vi "bit letters.vi"(8 "String \"0\"":string=" ", 9 "String \"1\"":string="#", 10 "Letras y string \"0\" / String \"1 y 0\"":bool=TRUE, 11 "Texto":string="Hola") -> (3 "big letters":string)   [LabVIEW 2019]
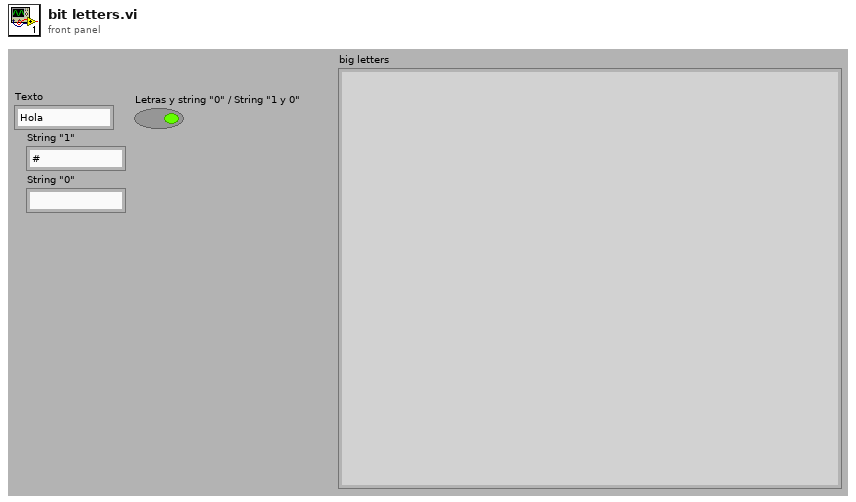
[diagram p1: front panel]
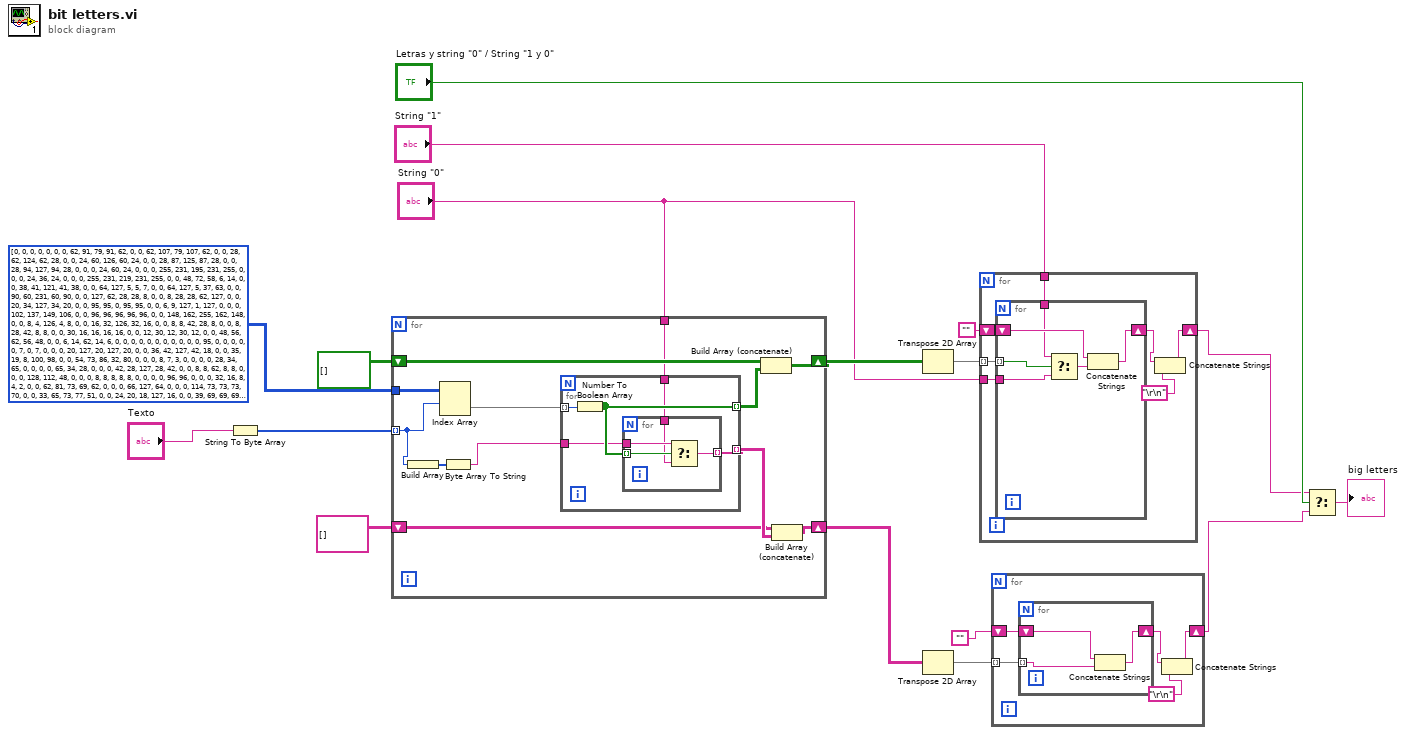
[diagram p0: block diagram]
diagram:
  n1 = String To Byte Array(string="Texto") -> (unsigned byte array=w16:u8[])
  n2 = for {
    tunnel: w16 -> [w24] mode=indexing
    tunnel: u8[][] [[0, 0, 0, 0, 0, 0, 0], [62, 91, 79, 91, 62, 0, 0], [62, 107, 79, 107, 62, 0, 0], [28, 62, 124, 62, 28, 0, 0], [24, 60, 126, 60, 24, 0, 0], [28, 87, 125, 87, 28, 0, 0], [28, 94, 127, 94, 28, 0, 0], [0, 24, 60, 24, 0, 0, 0], [255, 231, 195, 231, 255, 0, 0], [0, 24, 36, 24, 0, 0, 0], [255, 231, 219, 231, 255, 0, 0], [48, 72, 58, 6, 14, 0, 0], [38, 41, 121, 41, 38, 0, 0], [64, 127, 5, 5, 7, 0, 0], [64, 127, 5, 37, 63, 0, 0], [90, 60, 231, 60, 90, 0, 0], [127, 62, 28, 28, 8, 0, 0], [8, 28, 28, 62, 127, 0, 0], [20, 34, 127, 34, 20, 0, 0], [95, 95, 0, 95, 95, 0, 0], [6, 9, 127, 1, 127, 0, 0], [0, 102, 137, 149, 106, 0, 0], [96, 96, 96, 96, 96, 0, 0], [148, 162, 255, 162, 148, 0, 0], [8, 4, 126, 4, 8, 0, 0], [16, 32, 126, 32, 16, 0, 0], [8, 8, 42, 28, 8, 0, 0], [8, 28, 42, 8, 8, 0, 0], [30, 16, 16, 16, 16, 0, 0], [12, 30, 12, 30, 12, 0, 0], [48, 56, 62, 56, 48, 0, 0], [6, 14, 62, 14, 6, 0, 0], [0, 0, 0, 0, 0, 0, 0], [0, 0, 95, 0, 0, 0, 0], [0, 7, 0, 7, 0, 0, 0], [20, 127, 20, 127, 20, 0, 0], [36, 42, 127, 42, 18, 0, 0], [35, 19, 8, 100, 98, 0, 0], [54, 73, 86, 32, 80, 0, 0], [0, 8, 7, 3, 0, 0, 0], [0, 28, 34, 65, 0, 0, 0], [0, 65, 34, 28, 0, 0, 0], [42, 28, 127, 28, 42, 0, 0], [8, 8, 62, 8, 8, 0, 0], [0, 128, 112, 48, 0, 0, 0], [8, 8, 8, 8, 8, 0, 0], [0, 0, 96, 96, 0, 0, 0], [32, 16, 8, 4, 2, 0, 0], [62, 81, 73, 69, 62, 0, 0], [0, 66, 127, 64, 0, 0, 0], [114, 73, 73, 73, 70, 0, 0], [33, 65, 73, 77, 51, 0, 0], [24, 20, 18, 127, 16, 0, 0], [39, 69, 69, 69, 57, 0, 0], [60, 74, 73, 73, 49, 0, 0], [65, 33, 17, 9, 7, 0, 0], [54, 73, 73, 73, 54, 0, 0], [70, 73, 73, 41, 30, 0, 0], [0, 0, 20, 0, 0, 0, 0], [0, 64, 52, 0, 0, 0, 0], [0, 8, 20, 34, 65, 0, 0], [20, 20, 20, 20, 20, 0, 0], [0, 65, 34, 20, 8, 0, 0], [2, 1, 89, 9, 6, 0, 0], [62, 65, 93, 89, 78, 0, 0], [124, 18, 17, 18, 124, 0, 0], [127, 73, 73, 73, 54, 0, 0], [62, 65, 65, 65, 34, 0, 0], [127, 65, 65, 65, 62, 0, 0], [127, 73, 73, 73, 65, 0, 0], [127, 9, 9, 9, 1, 0, 0], [62, 65, 65, 81, 115, 0, 0], [127, 8, 8, 8, 127, 0, 0], [0, 65, 127, 65, 0, 0, 0], [32, 64, 65, 63, 1, 0, 0], [127, 8, 20, 34, 65, 0, 0], [127, 64, 64, 64, 64, 0, 0], [127, 2, 28, 2, 127, 0, 0], [127, 4, 8, 16, 127, 0, 0], [62, 65, 65, 65, 62, 0, 0], [127, 9, 9, 9, 6, 0, 0], [62, 65, 81, 33, 94, 0, 0], [127, 9, 25, 41, 70, 0, 0], [38, 73, 73, 73, 50, 0, 0], [3, 1, 127, 1, 3, 0, 0], [63, 64, 64, 64, 63, 0, 0], [31, 32, 64, 32, 31, 0, 0], [63, 64, 56, 64, 63, 0, 0], [99, 20, 8, 20, 99, 0, 0], [3, 4, 120, 4, 3, 0, 0], [97, 89, 73, 77, 67, 0, 0], [0, 127, 65, 65, 65, 0, 0], [2, 4, 8, 16, 32, 0, 0], [0, 65, 65, 65, 127, 0, 0], [4, 2, 1, 2, 4, 0, 0], [64, 64, 64, 64, 64, 0, 0], [0, 3, 7, 8, 0, 0, 0], [32, 84, 84, 120, 64, 0, 0], [127, 40, 68, 68, 56, 0, 0], [56, 68, 68, 68, 40, 0, 0], [56, 68, 68, 40, 127, 0, 0], [56, 84, 84, 84, 24, 0, 0], [0, 8, 126, 9, 2, 0, 0], [24, 164, 164, 156, 120, 0, 0], [127, 8, 4, 4, 120, 0, 0], [0, 68, 125, 64, 0, 0, 0], [32, 64, 64, 61, 0, 0, 0], [127, 16, 40, 68, 0, 0, 0], [0, 65, 127, 64, 0, 0, 0], [124, 4, 120, 4, 120, 0, 0], [124, 8, 4, 4, 120, 0, 0], [56, 68, 68, 68, 56, 0, 0], [252, 24, 36, 36, 24, 0, 0], [24, 36, 36, 24, 252, 0, 0], [124, 8, 4, 4, 8, 0, 0], [72, 84, 84, 84, 36, 0, 0], [4, 4, 63, 68, 36, 0, 0], [60, 64, 64, 32, 124, 0, 0], [28, 32, 64, 32, 28, 0, 0], [60, 64, 48, 64, 60, 0, 0], [68, 40, 16, 40, 68, 0, 0], [76, 144, 144, 144, 124, 0, 0], [68, 100, 84, 76, 68, 0, 0], [0, 8, 54, 65, 0, 0, 0], [0, 0, 119, 0, 0, 0, 0], [0, 65, 54, 8, 0, 0, 0], [2, 1, 2, 4, 2, 0, 0], [60, 38, 35, 38, 60, 0, 0], [30, 161, 161, 97, 18, 0, 0], [58, 64, 64, 32, 122, 0, 0], [56, 84, 84, 85, 89, 0, 0], [33, 85, 85, 121, 65, 0, 0], [33, 84, 84, 120, 65, 0, 0], [33, 85, 84, 120, 64, 0, 0], [32, 84, 85, 121, 64, 0, 0], [12, 30, 82, 114, 18, 0, 0], [57, 85, 85, 85, 89, 0, 0], [57, 84, 84, 84, 89, 0, 0], [57, 85, 84, 84, 88, 0, 0], [0, 0, 69, 124, 65, 0, 0], [0, 2, 69, 125, 66, 0, 0], [0, 1, 69, 124, 64, 0, 0], [240, 41, 36, 41, 240, 0, 0], [240, 40, 37, 40, 240, 0, 0], [124, 84, 85, 69, 0, 0, 0], [32, 84, 84, 124, 84, 0, 0], [124, 10, 9, 127, 73, 0, 0], [50, 73, 73, 73, 50, 0, 0], [50, 72, 72, 72, 50, 0, 0], [50, 74, 72, 72, 48, 0, 0], [58, 65, 65, 33, 122, 0, 0], [58, 66, 64, 32, 120, 0, 0], [0, 157, 160, 160, 125, 0, 0], [57, 68, 68, 68, 57, 0, 0], [61, 64, 64, 64, 61, 0, 0], [60, 36, 255, 36, 36, 0, 0], [72, 126, 73, 67, 102, 0, 0], [43, 47, 252, 47, 43, 0, 0], [255, 9, 41, 246, 32, 0, 0], [192, 136, 126, 9, 3, 0, 0], [32, 84, 84, 121, 65, 0, 0], [0, 0, 68, 125, 65, 0, 0], [48, 72, 72, 74, 50, 0, 0], [56, 64, 64, 34, 122, 0, 0], [0, 122, 10, 10, 114, 0, 0], [125, 13, 25, 49, 125, 0, 0], [38, 41, 41, 47, 40, 0, 0], [38, 41, 41, 41, 38, 0, 0], [48, 72, 77, 64, 32, 0, 0], [56, 8, 8, 8, 8, 0, 0], [8, 8, 8, 8, 56, 0, 0], [47, 16, 200, 172, 186, 0, 0], [47, 16, 40, 52, 250, 0, 0], [0, 0, 123, 0, 0, 0, 0], [8, 20, 42, 20, 34, 0, 0], [34, 20, 42, 20, 8, 0, 0], [170, 0, 85, 0, 170, 0, 0], [170, 85, 170, 85, 170, 0, 0], [0, 0, 0, 255, 0, 0, 0], [16, 16, 16, 255, 0, 0, 0], [20, 20, 20, 255, 0, 0, 0], [16, 16, 255, 0, 255, 0, 0], [16, 16, 240, 16, 240, 0, 0], [20, 20, 20, 252, 0, 0, 0], [20, 20, 247, 0, 255, 0, 0], [0, 0, 255, 0, 255, 0, 0], [20, 20, 244, 4, 252, 0, 0], [20, 20, 23, 16, 31, 0, 0], [16, 16, 31, 16, 31, 0, 0], [20, 20, 20, 31, 0, 0, 0], [16, 16, 16, 240, 0, 0, 0], [0, 0, 0, 31, 16, 0, 0], [16, 16, 16, 31, 16, 0, 0], [16, 16, 16, 240, 16, 0, 0], [0, 0, 0, 255, 16, 0, 0], [16, 16, 16, 16, 16, 0, 0], [16, 16, 16, 255, 16, 0, 0], [0, 0, 0, 255, 20, 0, 0], [0, 0, 255, 0, 255, 0, 0], [0, 0, 31, 16, 23, 0, 0], [0, 0, 252, 4, 244, 0, 0], [20, 20, 23, 16, 23, 0, 0], [20, 20, 244, 4, 244, 0, 0], [0, 0, 255, 0, 247, 0, 0], [20, 20, 20, 20, 20, 0, 0], [20, 20, 247, 0, 247, 0, 0], [20, 20, 20, 23, 20, 0, 0], [16, 16, 31, 16, 31, 0, 0], [20, 20, 20, 244, 20, 0, 0], [16, 16, 240, 16, 240, 0, 0], [0, 0, 31, 16, 31, 0, 0], [0, 0, 0, 31, 20, 0, 0], [0, 0, 0, 252, 20, 0, 0], [0, 0, 240, 16, 240, 0, 0], [16, 16, 255, 16, 255, 0, 0], [20, 20, 20, 255, 20, 0, 0], [16, 16, 16, 31, 0, 0, 0], [0, 0, 0, 240, 16, 0, 0], [255, 255, 255, 255, 255, 0, 0], [240, 240, 240, 240, 240, 0, 0], [255, 255, 255, 0, 0, 0, 0], [0, 0, 0, 255, 255, 0, 0], [15, 15, 15, 15, 15, 0, 0], [56, 68, 68, 56, 68, 0, 0], [124, 42, 42, 62, 20, 0, 0], [126, 2, 2, 6, 6, 0, 0], [2, 126, 2, 126, 2, 0, 0], [99, 85, 73, 65, 99, 0, 0], [56, 68, 68, 60, 4, 0, 0], [64, 126, 32, 30, 32, 0, 0], [6, 2, 126, 2, 2, 0, 0], [153, 165, 231, 165, 153, 0, 0], [28, 42, 73, 42, 28, 0, 0], [76, 114, 1, 114, 76, 0, 0], [48, 74, 77, 77, 48, 0, 0], [48, 72, 120, 72, 48, 0, 0], [188, 98, 90, 70, 61, 0, 0], [62, 73, 73, 73, 0, 0, 0], [126, 1, 1, 1, 126, 0, 0], [42, 42, 42, 42, 42, 0, 0], [68, 68, 95, 68, 68, 0, 0], [64, 81, 74, 68, 64, 0, 0], [64, 68, 74, 81, 64, 0, 0], [0, 0, 255, 1, 3, 0, 0], [224, 128, 255, 0, 0, 0, 0], [8, 8, 107, 107, 8, 0, 0], [54, 18, 54, 36, 54, 0, 0], [6, 15, 9, 15, 6, 0, 0], [0, 0, 24, 24, 0, 0, 0], [0, 0, 16, 16, 0, 0, 0], [48, 64, 255, 1, 1, 0, 0], [0, 31, 1, 1, 30, 0, 0], [0, 25, 29, 23, 18, 0, 0], [0, 60, 60, 60, 60, 0, 0], [0, 0, 0, 0, 0, 0, 0]] ("array") -> [w29]
    shift-right: [w26] -> w11
    shift-left: bool[][] [] -> [w27]
    shift-right: [w19] -> w9
    shift-left: string[][] [] -> [w20]
    tunnel: "String \"0\"" -> [w18]
    n3 = Build Array(w24) -> (w23:u8[])
    n4 = Index Array(array=w29, index (row)=w24) -> (element=w28:u8[])  [unwired: 1 in]
    n5 = Byte Array To String(unsigned byte array=w23) -> (string=w22:string)
    n6 = for {
      tunnel: w28 -> [w34] mode=indexing
      tunnel: [w33] -> w25 mode=indexing
      tunnel: w22 -> [w32]
      tunnel: [w31] -> w21 mode=indexing
      tunnel: w18 -> [w30]
      n7 = Number To Boolean Array(number=w34) -> (Boolean array=w33:bool[])
      n8 = for {
        tunnel: w33 -> [w38] mode=indexing
        tunnel: w32 -> [w37]
        tunnel: [w36] -> w31 mode=indexing
        tunnel: w30 -> [w35]
        n9 = Select(t=w37, s=w38, f=w35) -> (s? t:f=w36:string)
      }
    }
    n10 = Build Array (concatenate)(w27, w25) -> (w26:bool[][])
    n11 = Build Array (concatenate)(w20, w21) -> (w19:string[][])
  }
  n12 = Transpose 2D Array(2D array=w11) -> (transposed array=w13:bool[][])
  n13 = Transpose 2D Array(2D array=w9) -> (transposed array=w7:string[][])
  n14 = for {
    tunnel: w13 -> [w45] mode=indexing
    shift-right: [w41] -> w3
    shift-left: "" -> [w44]
    tunnel: "String \"1\"" -> [w40]
    tunnel: "String \"0\"" -> [w39]
    n15 = for {
      tunnel: w45 -> [w51] mode=indexing
      shift-right: [w48] -> w42
      shift-left: w44 -> [w50]
      tunnel: w40 -> [w47]
      tunnel: w39 -> [w46]
      n16 = Select(t=w47, s=w51, f=w46) -> (s? t:f=w49:string)
      n17 = Concatenate Strings(w50, w49) -> (w48:string)
    }
    n18 = Concatenate Strings(w42, "\r\n") -> (w41:string)
  }
  n19 = for {
    tunnel: w7 -> [w56] mode=indexing
    shift-right: [w52] -> w2
    shift-left: "" -> [w55]
    n20 = for {
      tunnel: w56 -> [w57] mode=indexing
      shift-right: [w58] -> w53
      shift-left: w55 -> [w59]
      n21 = Concatenate Strings(w59, w57) -> (w58:string)
    }
    n22 = Concatenate Strings(w53, "\r\n") -> (w52:string)
  }
  n23 = Select(t=w3, s="Letras y string \"0\" / String \"1 y 0\"", f=w2) -> (s? t:f=→"big letters":string)
